vi "GetSheetName.vi"(11 "String":string) -> (3 "whole match":string)   [LabVIEW 2014]
uses:
  <vilib>/regexp/Match Regular Expression.xnode
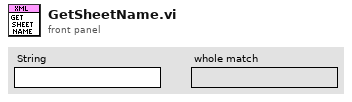
[diagram p1: front panel]
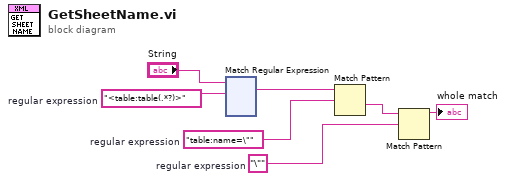
[diagram p0: block diagram]
diagram:
  w6 = "\""  # regular expression
  w4 = "table:name=\""  # regular expression
  w2 = "<table:table(.*?)>"  # regular expression
  n1 = xnode "Match Regular Expression"("input string"="String", "regular expression"=w2) -> ("whole match"=w3:string)  [unwired: 4 in, 4 out]
  n2 = Match Pattern(string=w3, regular expression=w4) -> (after substring=w5:string)  [unwired: 1 in, 3 out]
  n3 = Match Pattern(string=w5, regular expression=w6) -> (before substring=→"whole match":string)  [unwired: 1 in, 3 out]
